vi "gfitsio-write-column-boolean-1d.vi"(4 "units":string, 6 "row":i32, 7 "column":string, 8 "error in (no error)":errorcluster, 9 "data":bool[](array[boolean]), 10 "variable length? (T:yes)":bool=TRUE, 11 "gfits refnum":T1) -> (0 "error out":errorcluster, 3 "dup gfits refnum":T1)   [LabVIEW 2011, in "gfitsio.lvlib"]
doc: "Write data to the table column (doing data type conversion if necessary). This VI is not compatible with ASCII tables since ASCII tables can only contain scalar values columns."
uses:
  gfitsio.lvlib
  gfitsio-refnum.ctl
  cfitsio-hdutypes.ctl
  gfitsio.dll
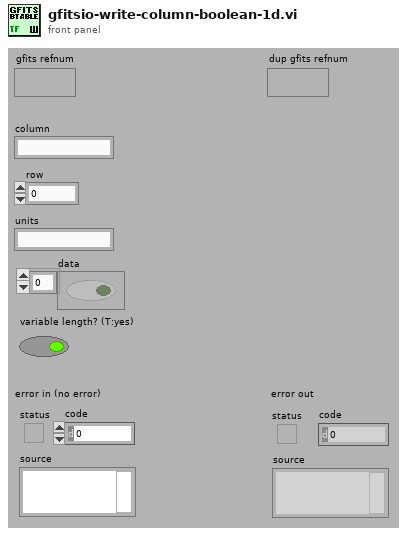
[diagram p1: front panel]
types:
  T1 = typedef "gfitsio.lvlib/gfitsio-refnum.ctl" = refnum<k1>
  T2 = typedef "gfitsio.lvlib/cfitsio-hdutypes.ctl" = i32
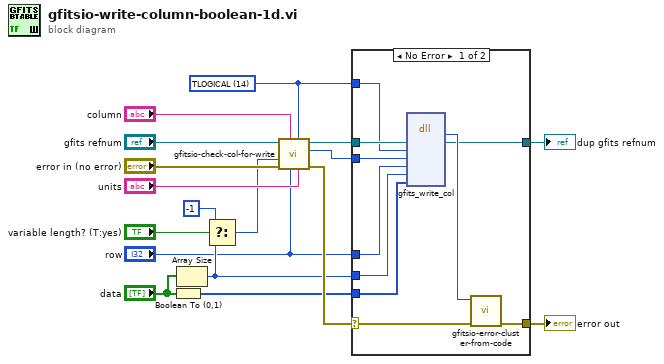
[diagram p0: block diagram]
diagram:
  w2 = T2 14 items=["TBIT"=1, "TBYTE  (U8)"=11, "TSBYTE  (I8)"=12, "TLOGICAL"=14, "TSTRING"=16, "TUSHORT  (U16)"=20, "TSHORT  (I16)"=21, "TUINT"=31, "TULONG  (U32)"=40, "TLONG  (I32)"=41, "TFLOAT  (SGL)"=42, "TLONGLONG  (I64)"=81, "TDOUBLE"=82, "TCOMPLEX  (CSG)"=83, "TDOUBLECOMPLEX  (CDB)"=163] ("cfitsio datatype")
  n1 = Boolean To (0,1)(Boolean="data") -> (0, 1=w1:i16[])
  n2 = Array Size(array="data") -> (size(s)=w6:i32)
  n3 = Select(t=-1, s="variable length? (T:yes)", f=w6) -> (s? t:f=w5:i32)
  n4 = call "gfitsio-check-col-for-write.vi"("units"="units", "cfitsio datatype"=w2, "row"="row", "column"="column", "error in (no error)"="error in (no error)", "size (-1:variable)"=w5, "gfits refnum"="gfits refnum") -> ("error out"=w11:errorcluster, "colnum"=w8:i32, "dup gfits refnum"=w13:T1)  [unwired: 2 in]
  n5 = case shown="No Error" w11 {
    selector: w11 -> [w27 w29]
    tunnel: [w26 w29] -> w16
    tunnel: w13 -> [w20 w28]
    tunnel: [w24 w28] -> w17
    tunnel: "row" -> [w23 _]
    tunnel: w1 -> [w22 _]
    tunnel: w8 -> [w21 _]
    tunnel: w6 -> [w19 _]
    tunnel: w2 -> [w18 _]
    frame No Error {
      n6 = dll-call lib="C:/BonOMM/BonOMM-SAOMM/SubVIs/gfitsio/gfitsio.dll" fn="gfits_write_col"("dup gfits refnum"=w20, "datatype"=w18, "column"=w21, "row"=w23, "nelements"=w19, "data"=w22) -> (w25:i32, "dup gfits refnum"=w24:T1)  [unwired: 8 in, 2 out]
      n7 = call "gfitsio-error-cluster-from-code.vi"("error in (no error)"=w27, "error code"=w25) -> ("error out"=w26:errorcluster)  [unwired: 9 in]
    }
    frame Error {
    }
  }
  "error out" <- w16
  "dup gfits refnum" <- w17
